vi "Read Aux Joystick V.3.0.vi"(11 "JoystickDevRef":T1) -> ()   [LabVIEW 2017]
uses:
  <vilib>/Rock Robotics/WPI/Joystick/WPI_JoystickDevRef.ctl
  <vilib>/Rock Robotics/WPI/Joystick/WPI_JoystickDeviceEnum.ctl
  Robot Global Data V.3.0.vi
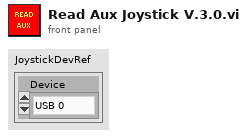
[diagram p1: front panel]
types:
  T1 = typedef "WPI_JoystickDevRef.ctl" = cluster{"Device":T2}
  T2 = typedef "WPI_JoystickDeviceEnum.ctl" = enum16{"USB 0", "USB 1", "USB 2", "USB 3", "USB 4", "USB 5"}
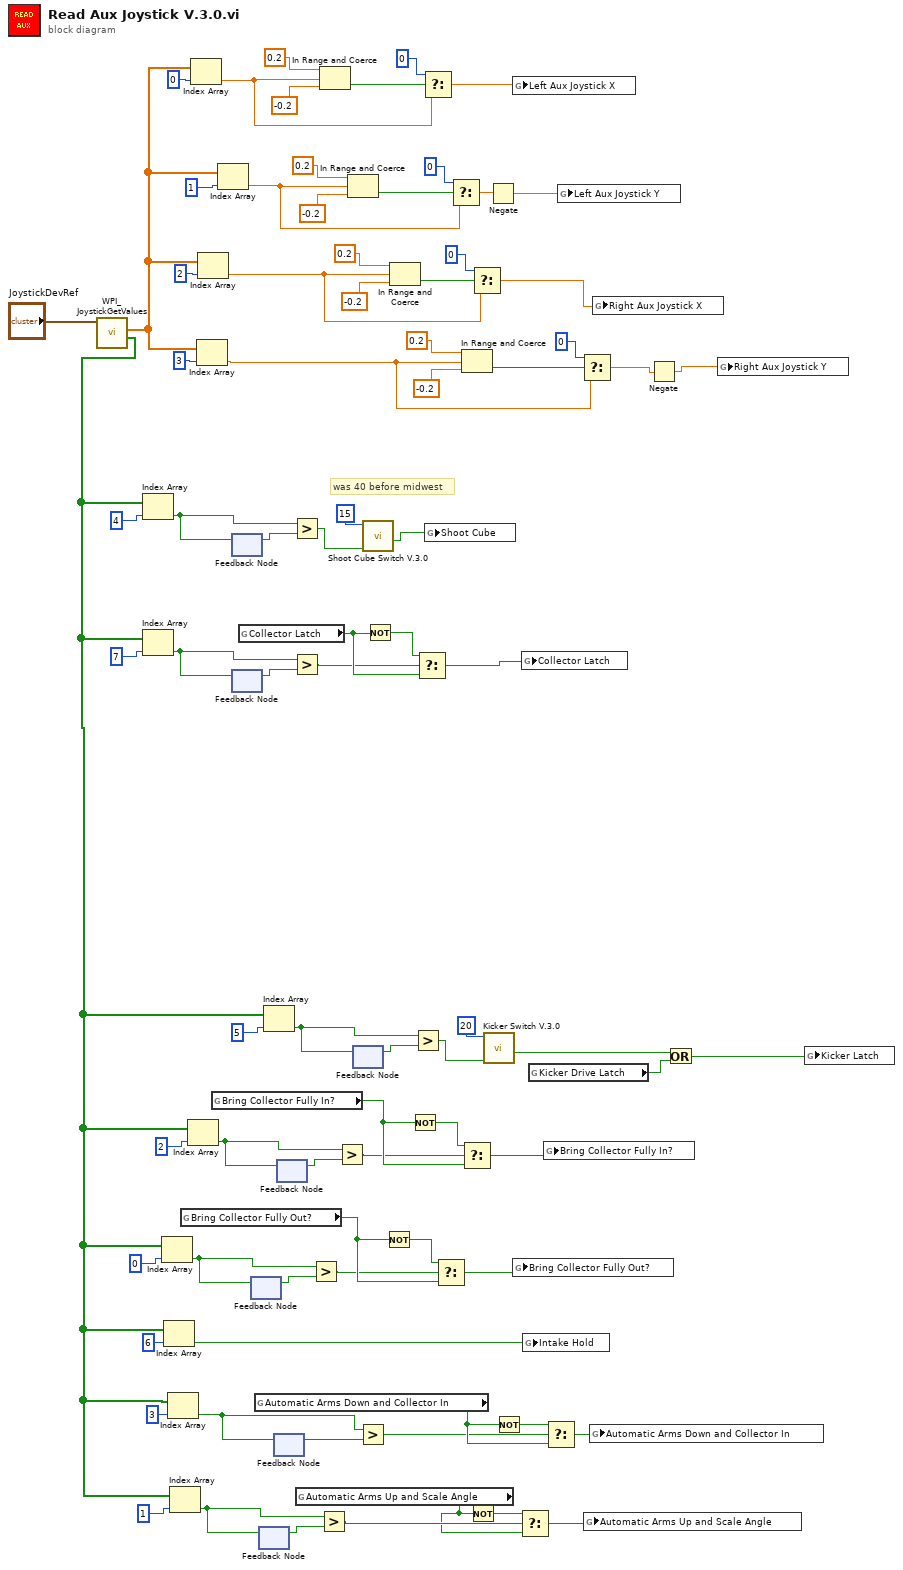
[diagram p0: block diagram]
diagram:
  # "was 40 before midwest"
  n1 = call <vilib>:"WPI_JoystickGetValues.vi"("JoystickDevRef"="JoystickDevRef") -> ("Buttons"=w1:bool[], "Axes"=w80:dbl[])  [unwired: 6 in, 3 out]
  n2 = Index Array(array=w1, index=4) -> (element=w50:bool)
  n3 = Index Array(array=w1, index=7) -> (element=w44:bool)
  n4 = Index Array(array=w1, index=0) -> (element=w25:bool)
  n5 = Index Array(array=w1, index=6) -> (element=w19:bool)
  n6 = Index Array(array=w1, index=3) -> (element=w9:bool)
  n7 = Index Array(array=w1, index=1) -> (element=w6:bool)
  n8 = global read "Robot Global Data V.3.0.vi" "Bring Collector Fully Out?"() -> (w23:bool)
  n9 = Index Array(array=w1, index=2) -> (element=w32:bool)
  n10 = Index Array(array=w80, index=0) -> (element=w75:dbl)
  n11 = Index Array(array=w80, index=3) -> (element=w53:dbl)
  n12 = Index Array(array=w80, index=2) -> (element=w65:dbl)
  n13 = global read "Robot Global Data V.3.0.vi" "Bring Collector Fully In?"() -> (w30:bool)
  n14 = Index Array(array=w80, index=1) -> (element=w70:dbl)
  n15 = feedback #1() -> (w51:bool)  [unwired: 1 in]
  n16 = feedback-in #1(w50) -> ()
  n17 = feedback #2() -> (w45:bool)  [unwired: 1 in]
  n18 = feedback-in #2(w44) -> ()
  n19 = global read "Robot Global Data V.3.0.vi" "Collector Latch"() -> (w42:bool)
  n20 = feedback #3() -> (w26:bool)  [unwired: 1 in]
  n21 = feedback-in #3(w25) -> ()
  n22 = global read "Robot Global Data V.3.0.vi" "Automatic Arms Down and Collector In"() -> (w12:bool)
  n23 = feedback #4() -> (w7:bool)  [unwired: 1 in]
  n24 = feedback-in #4(w6) -> ()
  n25 = Index Array(array=w1, index=5) -> (element=w37:bool)
  n26 = feedback #5() -> (w14:bool)  [unwired: 1 in]
  n27 = feedback-in #5(w9) -> ()
  n28 = feedback #6() -> (w33:bool)  [unwired: 1 in]
  n29 = feedback-in #6(w32) -> ()
  n30 = Greater?(x=w50, y=w51) -> (0:w48:bool)
  n31 = Greater?(x=w44, y=w45) -> (0:w40:bool)
  n32 = global read "Robot Global Data V.3.0.vi" "Automatic Arms Up and Scale Angle"() -> (w3:bool)
  n33 = Greater?(x=w25, y=w26) -> (0:w21:bool)
  n34 = Greater?(x=w6, y=w7) -> (0:w4:bool)
  n35 = In Range and Coerce(upper limit=0.2, x=w75, lower limit=-0.2) -> (In Range?=w77:bool)  [unwired: 1 out]
  n36 = Greater?(x=w32, y=w33) -> (0:w28:bool)
  n37 = In Range and Coerce(upper limit=0.2, x=w70, lower limit=-0.2) -> (In Range?=w72:bool)  [unwired: 1 out]
  n38 = feedback #7() -> (w38:bool)  [unwired: 1 in]
  n39 = feedback-in #7(w37) -> ()
  n40 = Greater?(x=w9, y=w14) -> (0:w11:bool)
  n41 = call "Shoot Cube Switch V.3.0.vi"("Input Button"=w48, "Time Until Reset"=15) -> ("On?"=w47:bool)  [unwired: 9 in]
  n42 = Not(x=w42) -> (.not. x?=w43:bool)
  n43 = Not(x=w23) -> (.not. x?=w24:bool)
  n44 = In Range and Coerce(upper limit=0.2, x=w65, lower limit=-0.2) -> (In Range?=w67:bool)  [unwired: 1 out]
  n45 = Not(x=w30) -> (.not. x?=w31:bool)
  n46 = Greater?(x=w37, y=w38) -> (0:w35:bool)
  n47 = Select(t=w43, s=w40, f=w42) -> (s? t:f=w41:bool)
  n48 = Select(t=0, s=w77, f=w75) -> (s? t:f=w57:dbl)
  n49 = global write "Robot Global Data V.3.0.vi" "Shoot Cube"(w47) -> ()
  n50 = Select(t=w24, s=w21, f=w23) -> (s? t:f=w22:bool)
  n51 = Select(t=0, s=w72, f=w70) -> (s? t:f=w60:dbl)
  n52 = In Range and Coerce(upper limit=0.2, x=w53, lower limit=-0.2) -> (In Range?=w62:bool)  [unwired: 1 out]
  n53 = Select(t=w31, s=w28, f=w30) -> (s? t:f=w29:bool)
  n54 = Not(x=w3) -> (.not. x?=w5:bool)
  n55 = Select(t=0, s=w67, f=w65) -> (s? t:f=w56:dbl)
  n56 = call "Kicker Switch V.3.0.vi"("Input Button"=w35, "Time Until Reset"=20) -> ("On?"=w18:bool)  [unwired: 9 in]
  n57 = Negate(x=w60) -> (-x=w55:dbl)
  n58 = Not(x=w12) -> (.not. x?=w13:bool)
  n59 = global write "Robot Global Data V.3.0.vi" "Left Aux Joystick X"(w57) -> ()
  n60 = global write "Robot Global Data V.3.0.vi" "Bring Collector Fully Out?"(w22) -> ()
  n61 = Select(t=w5, s=w4, f=w3) -> (s? t:f=w2:bool)
  n62 = global write "Robot Global Data V.3.0.vi" "Collector Latch"(w41) -> ()
  n63 = global write "Robot Global Data V.3.0.vi" "Intake Hold"(w19) -> ()
  n64 = global read "Robot Global Data V.3.0.vi" "Kicker Drive Latch"() -> (w17:bool)
  n65 = global write "Robot Global Data V.3.0.vi" "Bring Collector Fully In?"(w29) -> ()
  n66 = Select(t=w13, s=w11, f=w12) -> (s? t:f=w10:bool)
  n67 = global write "Robot Global Data V.3.0.vi" "Left Aux Joystick Y"(w55) -> ()
  n68 = Select(t=0, s=w62, f=w53) -> (s? t:f=w58:dbl)
  n69 = global write "Robot Global Data V.3.0.vi" "Automatic Arms Up and Scale Angle"(w2) -> ()
  n70 = global write "Robot Global Data V.3.0.vi" "Automatic Arms Down and Collector In"(w10) -> ()
  n71 = global write "Robot Global Data V.3.0.vi" "Right Aux Joystick X"(w56) -> ()
  n72 = Negate(x=w58) -> (-x=w59:dbl)
  n73 = Or(x=w18, y=w17) -> (x .or. y?=w16:bool)
  n74 = global write "Robot Global Data V.3.0.vi" "Right Aux Joystick Y"(w59) -> ()
  n75 = global write "Robot Global Data V.3.0.vi" "Kicker Latch"(w16) -> ()
